vi "Pixy Parser v.2.vi"() -> ()   [LabVIEW 2016]
panel:
  out "Objects Found":u16
  in  "Word in":u8[](array[numeric])
  out "Completed?":bool
  out "Frame Out":T1(array[cluster])
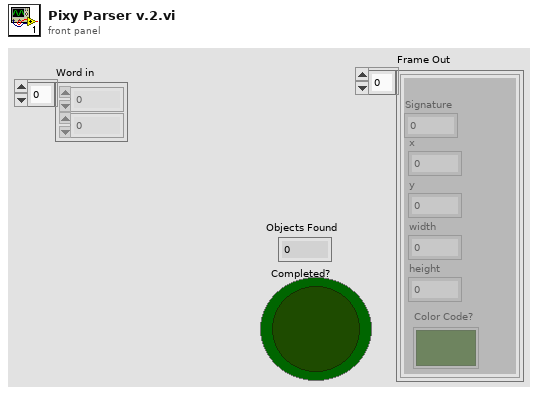
[diagram p1: front panel]
types:
  T1 = cluster{"x":u16, "y":u16, "width":u16, "height":u16, "Signature":u16, "Color Code?":bool}[]
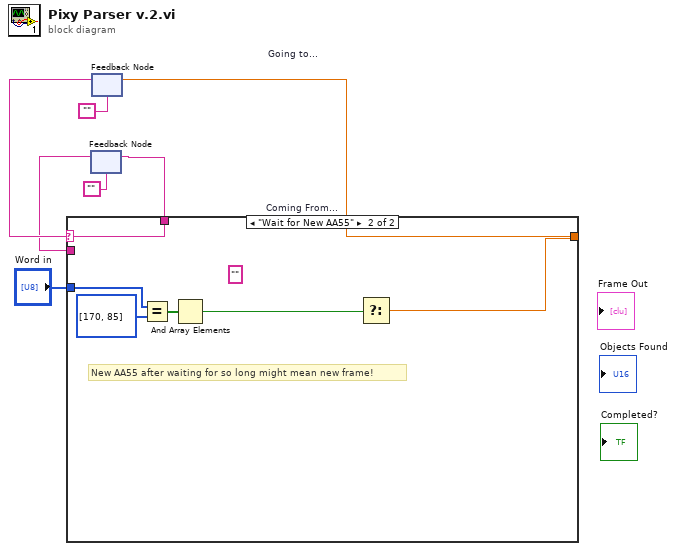
[diagram p0: block diagram]
diagram:
  n1 = feedback #1 "Coming From..."("") -> (w5:string)
  n2 = feedback #2 "Going to..."("") -> (w7:string)
  n3 = case shown="\"Wait for New AA55\"" w7 {
    selector: w7 -> [_ w13]
    tunnel: [_ w13] -> w6
    tunnel: w5 -> [_ _]
    tunnel: "Word in" -> [_ w12]
    tunnel: [_ w8] -> w3
    frame "\u0000", Default {
    }
    frame "Wait for New AA55" {
      (unwired) ""
      # "New AA55 after waiting for so long might mean new frame!"
      n4 = Equal?(x=w12, y=u8[] [170, 85]) -> (x = y?=w10:bool[])
      n5 = And Array Elements(Boolean array=w10) -> (logical AND=w9:bool)
      n6 = Select(s=w9) -> (s? t:f=w8:dbl)  [unwired: 2 in]
    }
  }
  n7 = feedback-in #1(w6) -> ()
  n8 = feedback-in #2(w3) -> ()
